vi "dare_Make_QRN.vi"(6 "AREF":T1, 8 "Q":T1, 9 "R":T1, 10 "B":T1, 11 "A":T1) -> (0 "Good":bool, 1 "N1":T1, 2 "R1":T1, 3 "Q1":T1)   [LabVIEW 2019]
uses:
  <vilib>/Analysis/Matrix/Datatypes/RealMatrix.ctl
  <vilib>/Analysis/baseanly.llb/Real A x B.vi
  <vilib>/Analysis/Matrix/Numeric/Add/Add - RM,RM.vi
  <vilib>/Analysis/Matrix/Numeric/Subtract/Subtract - RM,RM.vi
  <vilib>/Analysis/Matrix/NI_Matrix.lvlib
  <vilib>/Rock Robotics/WPI/ThirdParty/JAS_Junk/TrajLib/Trajectory_Library.lvlib
  <vilib>/Analysis/NI_AALBase.lvlib
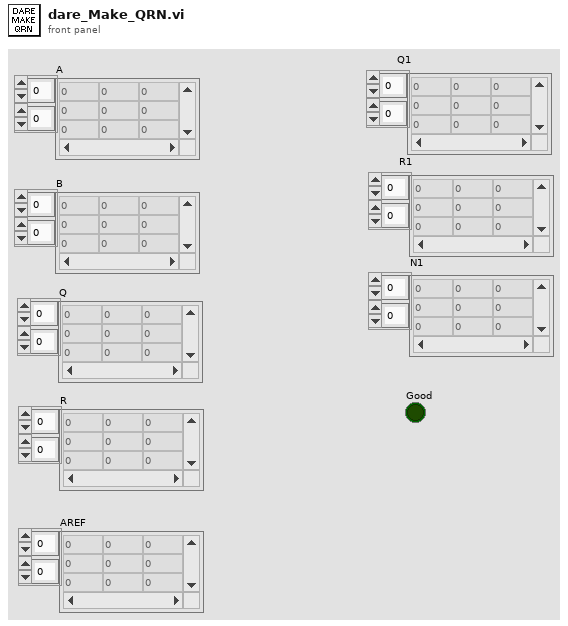
[diagram p1: front panel]
types:
  T1 = typedef "NI_Matrix.lvlib/RealMatrix.ctl" = dbl[][]
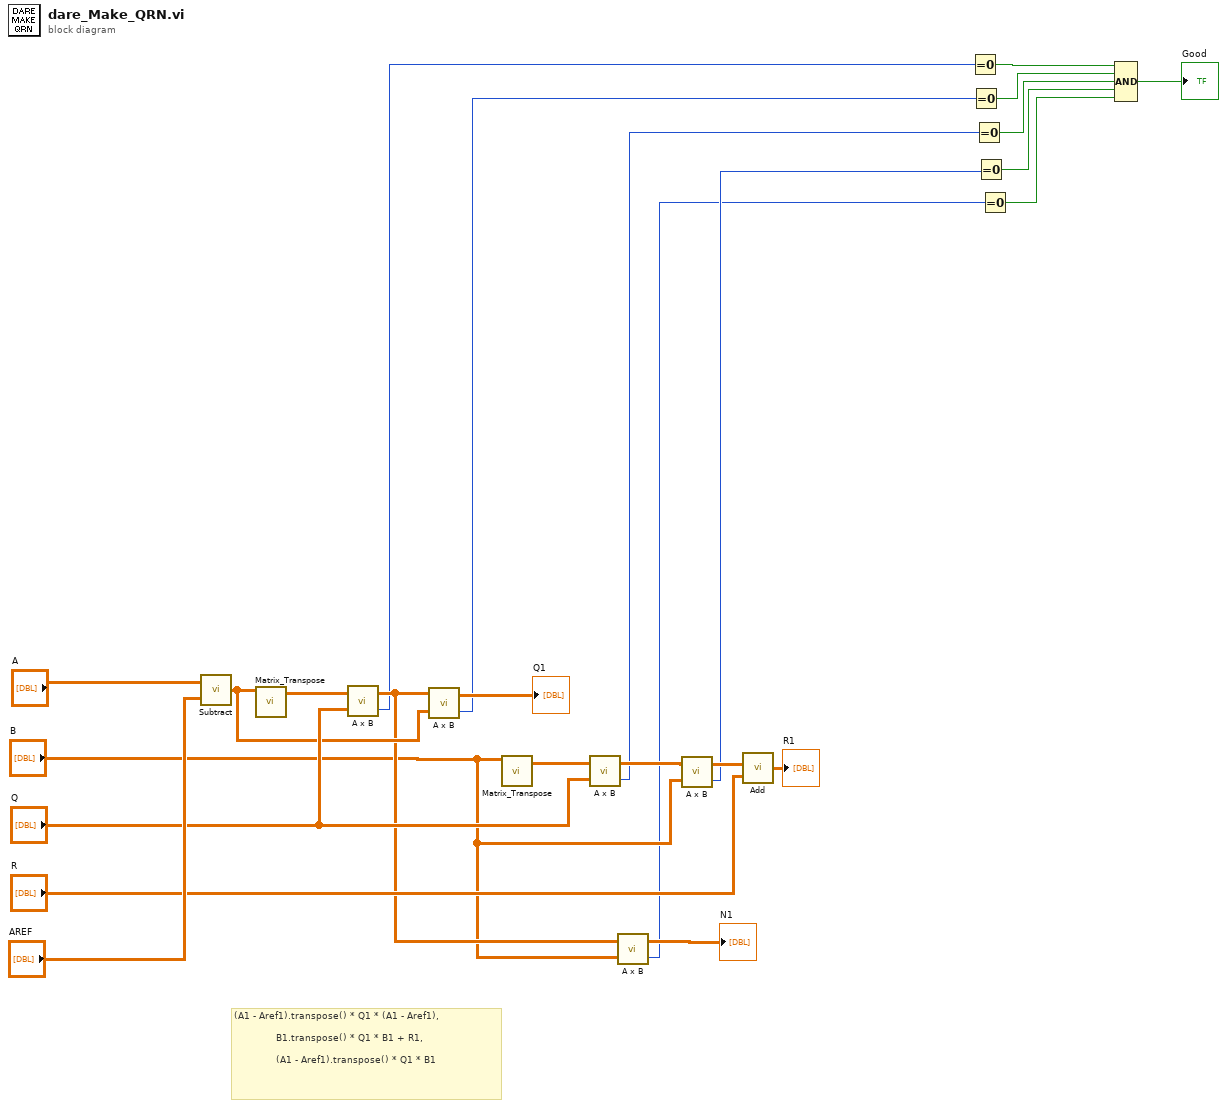
[diagram p0: block diagram]
diagram:
  # "(A1 - Aref1).transpose() * Q1 * (A1 - Aref1),\n\n              B1.transpose() * Q1 * B1 + R1,\n \n              (A1 - Aref1).transpose() * Q1 * B1"
  n1 = call-poly <vilib>:"Subtract.vi"("Real Matrix B"="AREF", "Real Matrix A"="A") -> ("A - B"=w12:T1)
  n2 = call <vilib>:"Matrix_Transpose.vi"("input matrix"=w12) -> ("output matrix"=w18:T1)  [unwired: 10 in]
  n3 = call-poly <vilib>:"A x B.vi"("B"="Q", "A"=w18) -> ("error"=w6:i32, "A x B"=w9:T1)
  n4 = call-poly <vilib>:"A x B.vi"("B"=w12, "A"=w9) -> ("error"=w5:i32, "A x B"=→"Q1":T1)
  n5 = call <vilib>:"Matrix_Transpose.vi"("input matrix"="B") -> ("output matrix"=w17:T1)  [unwired: 10 in]
  n6 = call-poly <vilib>:"A x B.vi"("B"="Q", "A"=w17) -> ("error"=w4:i32, "A x B"=w15:T1)
  n7 = call-poly <vilib>:"A x B.vi"("B"="B", "A"=w9) -> ("error"=w2:i32, "A x B"=→"N1":T1)
  n8 = call-poly <vilib>:"A x B.vi"("B"="B", "A"=w15) -> ("error"=w3:i32, "A x B"=w14:T1)
  n9 = call-poly <vilib>:"Add.vi"("Real Matrix B"="R", "Real Matrix A"=w14) -> ("A + B"=→"R1":T1)
  n10 = Equal To 0?(x=w6) -> (x = 0?=w21:bool)
  n11 = Equal To 0?(x=w5) -> (x = 0?=w22:bool)
  n12 = Equal To 0?(x=w4) -> (x = 0?=w23:bool)
  n13 = Equal To 0?(x=w3) -> (x = 0?=w24:bool)
  n14 = Equal To 0?(x=w2) -> (x = 0?=w25:bool)
  n15 = Compound Arithmetic op=AND(w21, w22, w23, w24, w25) -> (→"Good":bool)
